vi "SwitchDMM Channel UI.vi"() -> ()   [LabVIEW 2025, in "SwitchDMM Channel.lvclass"]
doc: "Copyright 2017 National Instruments Corporation\n\nLicensed under the Apache License, Version 2.0 (the \"License\"); you may not use this file except in compliance with the License. You may obtain a copy of the License at http://www.apache.org/licenses/LICENSE-2.0\nUnless required by applicable law or agreed to in writing, software distributed under the License is distributed on an \"AS IS\" BASIS, WITHOUT WARRANTIES OR CONDITIONS OF ANY KIND, either express or implied. See the License for the specific language governing permissions and limitations under the License."
uses:
  SwitchDMM Channel.lvclass
  Users/Public/Documents/Sandia National Labs/TSS Plugin/CEF.lvlibp/Node/NodeRef.ctl
  Users/Public/Documents/Sandia National Labs/TSS Plugin/CEF.lvlibp/Node/CEF_Node.lvclass
  Users/Public/Documents/Sandia National Labs/TSS Plugin/CEF.lvlibp/Node/mainQref.ctl
  Users/Public/Documents/Sandia National Labs/TSS Plugin/CEF.lvlibp/Node/UserEventRef.ctl
  Users/Public/Documents/Sandia National Labs/TSS Plugin/Abstract Engine.lvlibp/Plugin/Abstract/Channel configuration/Default Channel.ctl
  SwitchDMM Channel configuration/SwitchDMM Channel.ctl
  C:/Users/Public/Documents/Sandia National Labs/TSS Plugin/CEF.lvlibp/Node/CEF_Node.lvclass
  DMM Instrument/DMM Instrument.lvclass
  SwitchDMM Channel.lvclass/SwitchDMM Channel.ctl
  SwitchDMM Channel configuration/SwitchDMM Channel configuration.lvclass/SwitchDMM Channel configuration.ctl
  SwitchDMM Channel configuration/Read SwitchDMM Channel.vi
  SwitchDMM Channel configuration/Write SwitchDMM Channel.vi
  <vilib>/Utility/error.llb/Trim Whitespace One-Sided.vi
  SwitchDMM Channel configuration/SwitchDMM Channel configuration.lvclass
  C:/Users/Public/Documents/Sandia National Labs/TSS Plugin/Abstract Engine.lvlibp/Plugin/Abstract/Channel configuration/Channel configuration.lvclass
  Users/Public/Documents/Sandia National Labs/TSS Plugin/CEF.lvlibp/Node/ReadParent.vi
  Users/Public/Documents/Sandia National Labs/TSS Plugin/Abstract Engine.lvlibp/Plugin/Abstract/Channel configuration/Read Channel Setting.vi
  Users/Public/Documents/Sandia National Labs/TSS Plugin/Abstract Engine.lvlibp/Plugin/Abstract/Channel configuration/Write Channel Setting.vi
  Users/Public/Documents/Sandia National Labs/TSS Plugin/CEF.lvlibp
  Users/Public/Documents/Sandia National Labs/TSS Plugin/Abstract Engine.lvlibp/Plugin/Abstract/Abstract Engine/Abstract Engine.lvclass
  Users/Public/Documents/Sandia National Labs/TSS Plugin/Abstract Engine.lvlibp/Plugin/Abstract/Channel configuration/Channel configuration.lvclass
panel:
  in  "DMM Channel":cluster{"Default":T1, "Setting":T2}={"Default"={"Address"="localhost", "SW Alias"="ch0", "Enabled"=TRUE, "Type"="None", "Description"=""}, "Setting"={"Switch"="com0->ch0"}}
  in  "user event":T3
  in  "main queue":T4
  in  "node ref":T5
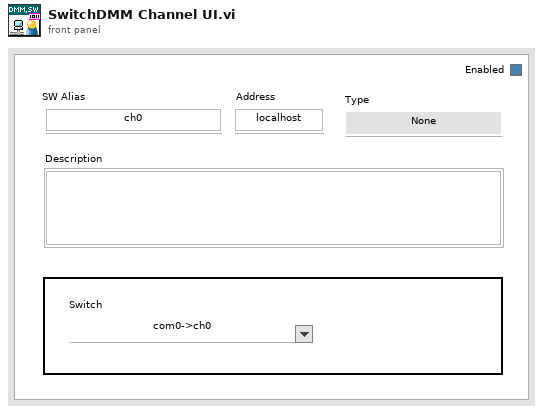
[diagram p1: front panel]
types:
  T1 = typedef "Abstract Engine.lvlibp/Channel configuration.lvclass/Default Channel.ctl" = cluster{"Address":string, "SW Alias":string, "Enabled":bool, "Type":string, "Description":string}
  T2 = typedef "SwitchDMM Channel configuration.lvclass/SwitchDMM Channel.ctl" = cluster{"Switch":string}
  T3 = typedef "CEF.lvlibp/CEF_Node.lvclass/UserEventRef.ctl" = refnum<user-event>
  T4 = typedef "CEF.lvlibp/CEF_Node.lvclass/mainQref.ctl" = refnum<queue>
  T5 = typedef "CEF.lvlibp/CEF_Node.lvclass/NodeRef.ctl" = refnum<data-value>
  T6 = cluster{"Channel Setting":T1, "SwitchDMM Channel":T2}
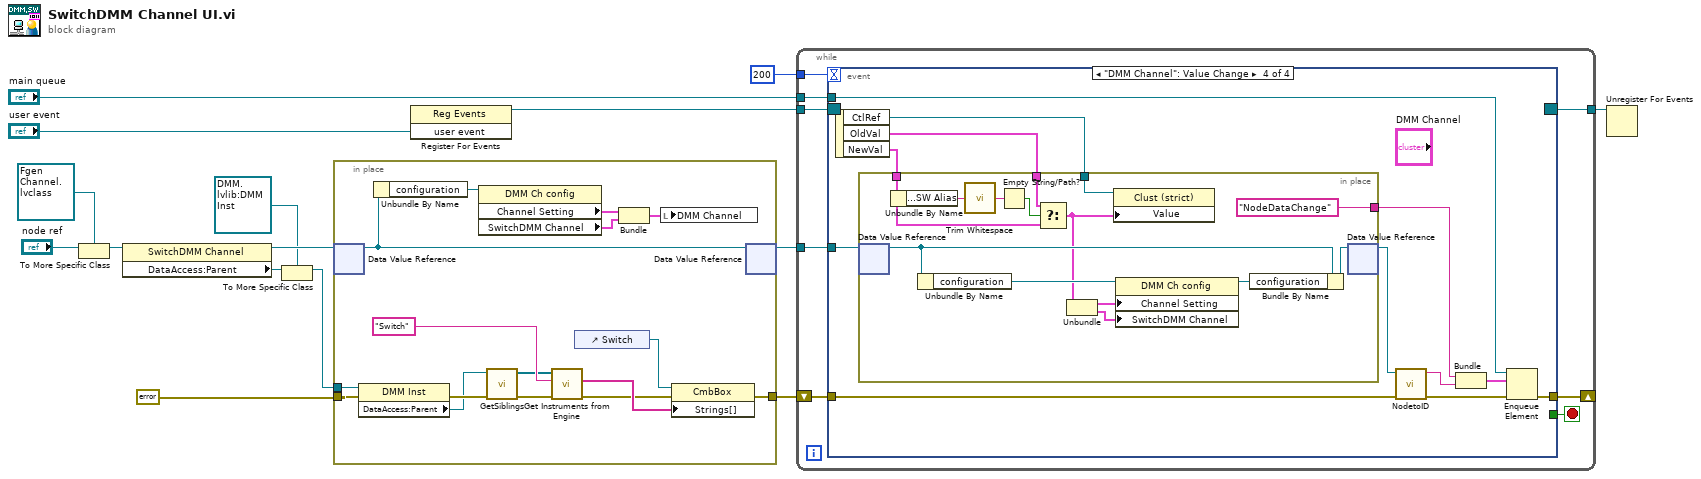
[diagram p0: block diagram]
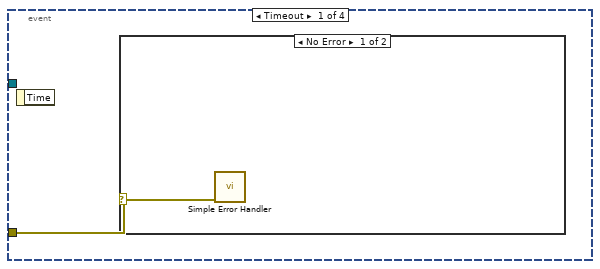
[diagram p2: hidden frame]
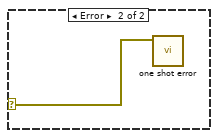
[diagram p3: hidden frame]
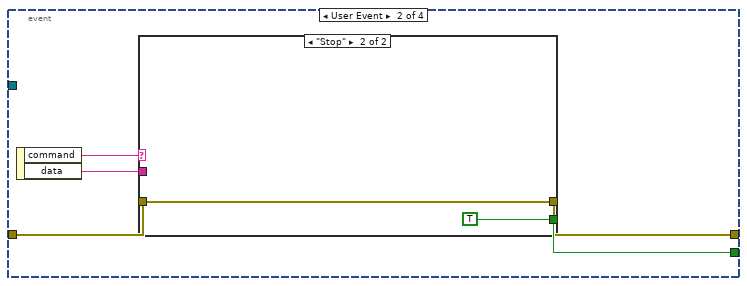
[diagram p4: hidden frame]
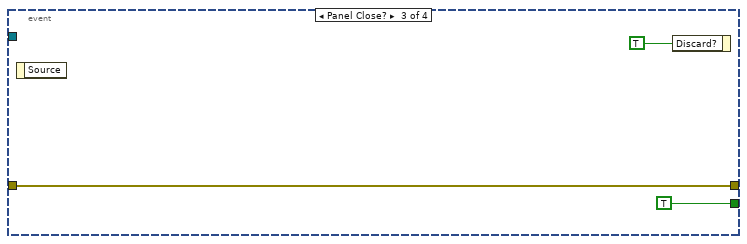
[diagram p6: hidden frame]
diagram:
  n1 = To More Specific Class(target class=refnum<data-value> refnum ("data value reference"), reference="node ref") -> (specific class reference=w6:refnum<data-value>)  [unwired: 1 in, 1 out]
  n2 = property class="SwitchDMM Channel"(reference=w6) -> (reference out=w4:refnum<data-value>, "DataAccess:Parent"=w3:refnum<data-value>)  [unwired: 1 in, 1 out]
  n3 = To More Specific Class(target class=refnum<data-value> refnum ("data value reference"), reference=w3) -> (specific class reference=w1:refnum<data-value>)  [unwired: 1 in, 1 out]
  n4 = in-place {
    in-place-border: errorcluster {"status"=FALSE, "code"=0, "source"=""} ("error out") -> [w21]
    in-place-border: [w27] -> w5
    in-place-border: w1 -> [w22]
    # "Initialize the front panel controls when loaded"
    n5 = in-place-dvr #1(w4) -> (w26:refnum<class "SwitchDMM Channel.lvclass">)  [unwired: 1 out]
    n6 = property class="DMM Inst"(reference=w22, error in=w21) -> (error out=w20:errorcluster, "DataAccess:Parent"=w17:refnum<data-value>)  [unwired: 1 out]
    n7 = Unbundle By Name(w26) -> ("configuration"=w31:refnum<class "SwitchDMM Channel configuration.lvclass">)
    n8 = property class="DMM Ch config"(reference=w31) -> ("Channel Setting"=w30:T1, "SwitchDMM Channel"=w29:T2)  [unwired: 1 in, 2 out]
    n9 = call "GetSiblings.vi"("error in"=w20, "node in"=w17) -> ("error out"=w18:errorcluster, "siblings"=w16:refnum<data-value>[])  [unwired: 8 in]
    n10 = call "Get Instruments from Engine.vi"("error in"=w18, "Engine"="Switch", "Engines"=w16) -> ("error out"=w23:errorcluster, "Instruments"=w24:string[])  [unwired: 6 in, 1 out]
    n11 = control-ref of="Switch"() -> (w19:refnum<vi>)
    n12 = Bundle("Channel Setting"=w30, "SwitchDMM Channel"=w29) -> (w28:T6)  [unwired: 1 in]
    n13 = local write "DMM Channel"(w28) -> ()
    n14 = property class="CmbBox"(reference=w19, error in=w23, "Strings[]"=w24) -> (error out=w27:errorcluster)  [unwired: 1 out]
    n15 = in-place-dvr #1(w26) -> (w9:refnum<data-value>)  [unwired: 1 out]
  }
  n16 = register-events("user event") -> (reference out=w14:refnum<event-registration>)  [unwired: 2 in, 1 out]
  n17 = while {
    tunnel: w9 -> [w39]
    tunnel: w14 -> [w38]
    tunnel: [w37] -> w13
    shift-right: [w34] -> _
    shift-left: w5 -> [w36]
    tunnel: "main queue" -> [w33]
    tunnel: 200 -> [w32]
    stop <- w35 stop-if-true
    n18 = event shown="[3] \"DMM Channel\": Value Change" {
      selector: w38 -> [_ _ _ _]
      dyn-events: [_ _ _ _] -> w37
      timeout: w32 -> [_ _ _ _]
      tunnel: w39 -> [_ _ _ w63]
      tunnel: [_ w43 w51 w64] -> w34
      tunnel: w36 -> [w40 w44 w51 w56]
      tunnel: [_ w47 TRUE _] -> w35
      tunnel: w33 -> [_ _ _ w65]
      event Timeout {
        n19 = event-data() -> ()  [unwired: 1 in, 1 out]
        n20 = case shown="No Error" w40 {
          selector: w40 -> [w41 w42]
          frame No Error {
            n21 = call <vilib>:"Simple Error Handler.vi"("error in (no error)"=w41) -> ()  [unwired: 4 in, 5 out]
          }
          frame Error {
            n22 = call "one shot error.vi"("error in"=w42) -> ()  [unwired: 11 in]
          }
        }
      }
      event User Event {
        n23 = event-data() -> ("command"=w45:string, "data"=w46:string)  [unwired: 1 in]
        n24 = case shown="\"Stop\"" w45 {
          tunnel: w46 -> [_ _]
          tunnel: [_ TRUE] -> w47
          tunnel: w44 -> [w48 w49]
          tunnel: [w48 w49] -> w43
          frame Default {
          }
          frame "Stop" {
          }
        }
      }
      event Panel Close? {
        n25 = event-data() -> ()  [unwired: 1 in, 1 out]
        n26 = event-data("Discard?"=TRUE) -> ()  [unwired: 1 in, 1 out]
      }
      event "DMM Channel": Value Change {
        n27 = event-data() -> ("CtlRef"=w60:refnum<vi>, "OldVal"=w61:cluster{"Default":T1, "Setting":T2}, "NewVal"=w59:cluster{"Default":T1, "Setting":T2})  [unwired: 1 in]
        n28 = in-place {
          in-place-border: w61 -> [w75]
          in-place-border: w59 -> [w72]
          in-place-border: w60 -> [w74]
          in-place-border: ["NodeDataChange" ("Message Name")] -> w58
          n29 = in-place-dvr #2(w63) -> (w79:refnum<class "SwitchDMM Channel.lvclass">)  [unwired: 1 out]
          n30 = Unbundle By Name(w72) -> ("Default.SW Alias"=w73:string)
          n31 = Unbundle By Name(w79) -> ("configuration"=w77:refnum<class "SwitchDMM Channel configuration.lvclass">)
          n32 = call <vilib>:"Trim Whitespace.vi"("string"=w73) -> ("trimmed string"=w70:string)  [unwired: 1 in]
          n33 = Empty String/Path?(string/path=w70) -> (empty?=w71:bool)
          n34 = Select(t=w75, s=w71, f=w72) -> (s? t:f=w68:cluster{"Default":T1, "Setting":T2})
          n35 = Unbundle(w68) -> ("Default"=w67:T1, "Setting"=w66:T2)
          n36 = property class="Clust (strict)"(reference=w74, "Value"=w68) -> ()  [unwired: 1 in, 2 out]
          n37 = property class="DMM Ch config"(reference=w77, "Channel Setting"=w67, "SwitchDMM Channel"=w66) -> (reference out=w76:refnum<class "SwitchDMM Channel configuration.lvclass">)  [unwired: 1 in, 1 out]
          n38 = Bundle By Name(cluster=w79, "configuration"=w76) -> (w78:refnum<class "SwitchDMM Channel.lvclass">)
          n39 = in-place-dvr #2(w78) -> (w62:refnum<data-value>)  [unwired: 1 out]
        }
        n40 = call "NodetoID.vi"("error in"=w56, "node ref"=w62) -> ("error out"=w55:errorcluster, "ID"=w57:string)  [unwired: 8 in]
        n41 = Bundle("Message Name"=w58, "ID"=w57) -> (w54:cluster{"Message Name":string, "ID":string})  [unwired: 1 in]
        n42 = Enqueue Element(queue=w65, element=w54, error in (no error)=w55) -> (error out=w64:errorcluster)  [unwired: 1 in, 2 out]
      }
    }
  }
  n43 = Unregister For Events(event registration refnum=w13) -> ()  [unwired: 1 in, 1 out]
